vi "test_RLBoat.vi"() -> ()   [LabVIEW 2020]
uses:
  <vilib>/Instr/_visa.llb/VISA Configure Serial Port (Instr).vi
panel:
  in  "speed r":u8(slide)=100 scale=104.0..150.0
  in  "port":refnum<visa-resource-name>="COM9"
  in  "rate":u32=115200
  in  "stop":bool
  out "String":string="spl=28,st=28,dir=b,light=0,spr=28,\r\n"
  out "write buffer":string="28,28,b,0,SRC 2021-05-30 오후 12:16:22,28, &"
  in  "speed l":i16(slide)=100 scale=104.0..150.0
  in  "steer":i16(slide)=28 scale=0.0..35.0
  in  "M dir":bool
  in  "Led":bool
  in  "msg":string="SRC "
  in  "Write":bool=TRUE
  out "seriai R buff Chart":u32(graph)=36
  out "N":i32=50
  out "read buffer":string="spl=28,st=28,dir=b,light=0,spr=28,\r\n"
  out "steer servo":i32(knob)=28 scale=15.0..35.0
  out "seriai R feedback":cluster{i32, i32}(graph)={28, 28}
  in  "dt":u32=50
  # "Arduino ESC Control"
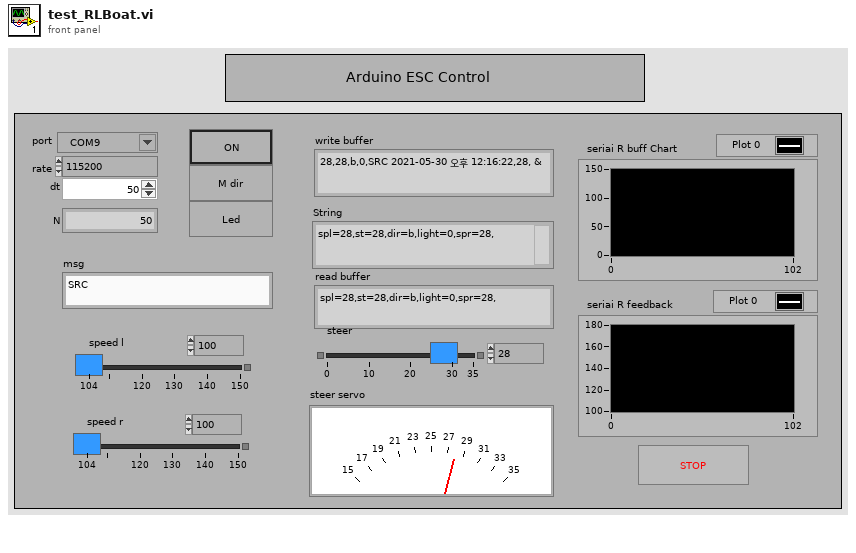
[diagram p1: front panel]
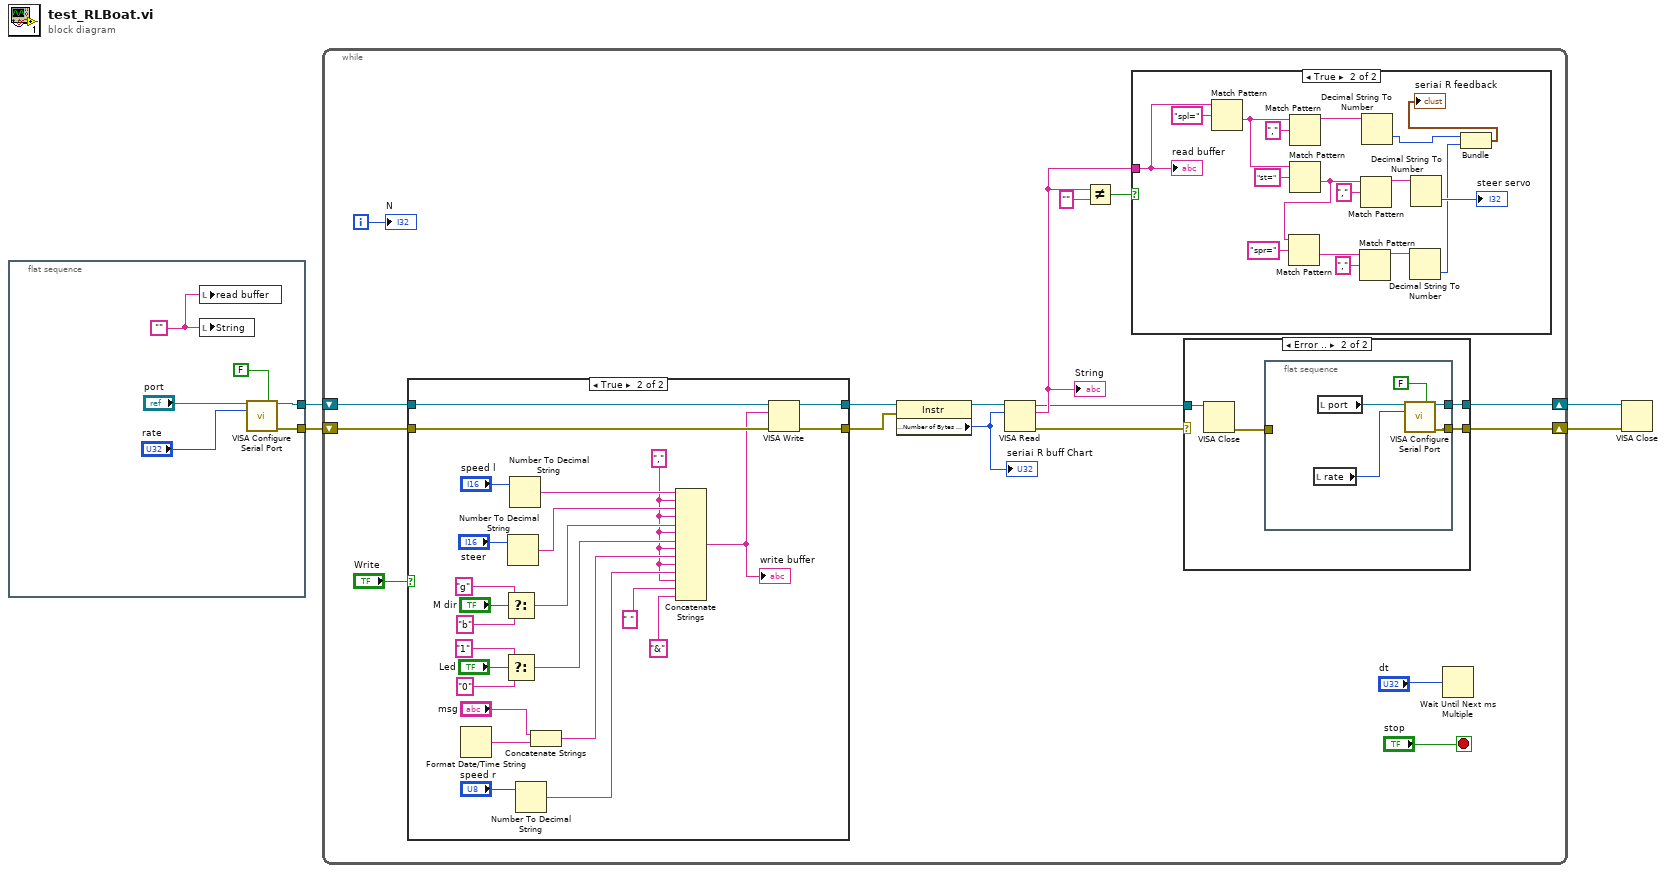
[diagram p0: block diagram]
diagram:
  n1 = flat-sequence {
    tunnel: [w9] -> w4
    tunnel: [w8] -> w1
    frame #0 {
      w5 = ""
      n2 = local write "read buffer"(w5) -> ()
      n3 = local write "String"(w5) -> ()
      n4 = call-poly "VISA Configure Serial Port"("port"="port", "Enable Termination\nChar (T)"=FALSE ("Enable Termination\nChar (T)"), "baud rate (9600)"="rate") -> ("port out"=w9:refnum<visa-resource-name>, "error out"=w8:errorcluster)  [unwired: 11 in]
    }
  }
  n5 = while {
    shift-right: [w11] -> w3
    shift-left: w4 -> [w27]
    shift-right: [w12] -> w2
    shift-left: w1 -> [w26]
    i -> [w19]
    stop <- "stop" stop-if-true
    n6 = case shown="True" "Write" {
      tunnel: w27 -> [w57 w82]
      tunnel: [w56 w81] -> w20
      tunnel: w26 -> [w56 w80]
      tunnel: [w57 w79] -> w22
      frame False {
      }
      frame True {
        w58 = "," ("string")
        n7 = Format Date/Time String() -> (date/time string=w63:string)  [unwired: 3 in]
        n8 = Select(t="g" ("string"), s="M dir", f="b" ("string")) -> (s? t:f=w69:string)
        n9 = Select(t="1" ("string"), s="Led", f="0" ("string")) -> (s? t:f=w65:string)
        n10 = Number To Decimal String(number="steer") -> (decimal integer string=w73:string)  [unwired: 1 in]
        n11 = Number To Decimal String(number="speed l") -> (decimal integer string=w77:string)  [unwired: 1 in]
        n12 = Number To Decimal String(number="speed r") -> (decimal integer string=w59:string)  [unwired: 1 in]
        n13 = Concatenate Strings("msg", w63) -> (w61:string)
        n14 = Concatenate Strings(w77, w58, w73, w58, w69, w58, w65, w58, w61, w58, w59, w58, " " ("문자열"), "&" ("string")) -> (w75:string)
        "write buffer" <- w75
        n15 = VISA Write(VISA resource name=w82, write buffer=w75, error in (no error)=w80) -> (VISA resource name out=w79:refnum<visa-resource-name>, error out=w81:errorcluster)  [unwired: 1 out]
      }
    }
    n16 = property class="Instr"(reference=w22, error in=w20) -> (reference out=w23:refnum<visa-resource-name>, "Serial Settings:Number of Bytes at Serial Port"=w18:u32)  [unwired: 1 out]
    "seriai R buff Chart" <- w18
    n17 = VISA Read(VISA resource name=w23, byte count=w18) -> (VISA resource name out=w13:refnum<visa-resource-name>, read buffer=w15:string, error out=w14:errorcluster)  [unwired: 1 in, 1 out]
    "String" <- w15
    n18 = Not Equal?(x=w15, y="") -> (x != y?=w16:bool)
    n19 = case shown="True" w16 {
      tunnel: w15 -> [_ w55]
      frame False {
      }
      frame True {
        n20 = Match Pattern(string=w55, regular expression="spl=" ("정규식")) -> (after substring=w48:string)  [unwired: 1 in, 3 out]
        n21 = Match Pattern(string=w48, regular expression="," ("정규식")) -> (before substring=w52:string)  [unwired: 1 in, 3 out]
        n22 = Match Pattern(string=w48, regular expression="st=" ("정규식")) -> (after substring=w42:string)  [unwired: 1 in, 3 out]
        n23 = Match Pattern(string=w42, regular expression="spr=" ("정규식")) -> (after substring=w46:string)  [unwired: 1 in, 3 out]
        n24 = Match Pattern(string=w46, regular expression="," ("정규식")) -> (before substring=w43:string)  [unwired: 1 in, 3 out]
        n25 = Match Pattern(string=w42, regular expression="," ("정규식")) -> (before substring=w51:string)  [unwired: 1 in, 3 out]
        n26 = Decimal String To Number(string=w52) -> (number=w40:i32)  [unwired: 2 in, 1 out]
        n27 = Decimal String To Number(string=w43) -> (number=w41:i32)  [unwired: 2 in, 1 out]
        n28 = Decimal String To Number(string=w51) -> (number=→"steer servo":i32)  [unwired: 2 in, 1 out]
        n29 = Bundle(w40, w41) -> (→"seriai R feedback":cluster{i32, i32})  [unwired: 1 in]
        "read buffer" <- w55
      }
    }
    n30 = case shown="Error .." w14 {
      selector: w14 -> [w28 _]
      tunnel: w13 -> [w29 w33]
      tunnel: [w28 w31] -> w12
      tunnel: [w29 w30] -> w11
      frame No Error {
      }
      frame Error {
        n31 = VISA Close(VISA resource name=w33) -> (error out=w32:errorcluster)  [unwired: 1 in]
        n32 = flat-sequence {
          tunnel: w32 -> [_]
          tunnel: [w35] -> w31
          tunnel: [w34] -> w30
          frame #0 {
            n33 = local read "rate"() -> (w36:u32)
            n34 = local read "port"() -> (w37:refnum<visa-resource-name>)
            n35 = call-poly "VISA Configure Serial Port"("port"=w37, "Enable Termination\nChar (T)"=FALSE ("Enable Termination\nChar (T)"), "baud rate (9600)"=w36) -> ("port out"=w34:refnum<visa-resource-name>, "error out"=w35:errorcluster)  [unwired: 11 in]
          }
        }
      }
    }
    n36 = Wait Until Next ms Multiple(millisecond multiple="dt") -> ()  [unwired: 1 out]
    "N" <- w19
  }
  n37 = VISA Close(VISA resource name=w3, error in (no error)=w2) -> ()  [unwired: 1 out]
